vi "Stop Core.vi"(10 "final error code":i32, 11 "Device in":refnum<class "Device.lvclass">) -> (3 "Device out":refnum<class "Device.lvclass">)   [LabVIEW 2014, in "DAQ Device.lvlib" / "Device.lvclass"]
doc: "(<B>Filename</B>: Actor Framework.lvlib:Actor.lvclass:Stop Core.vi)\n\nDefines what the actor does before it stops. Use the <B>final error code</B> input to determine whether the actor shut down in response to an error.\n\nBy default, this method does nothing. A descendant class may override it to define behavior, such as shutting down any processes the actor initiated in its override of the Actor Core method."
uses:
  Device.lvclass
  SuperActor/SuperActor.lvclass/SuperActor.ctl
  Device.lvclass/Device.ctl
  SuperActor/Read Log Session.vi
  SuperActor/Read ID.vi
  <userlib>/_Session Fwk/Session - Root.lvclass
  Devices/Configurable Device/Configurable Device.lvclass
  SuperActor/SuperActor.lvclass
  Session APIs/Session Log/System Log.lvclass
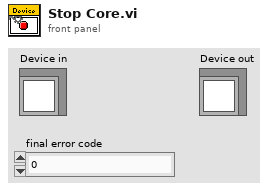
[diagram p1: front panel]
types:
  T1 = typedef "Session - Root.lvclass/Session Handle.ctl" = refnum<data-value>
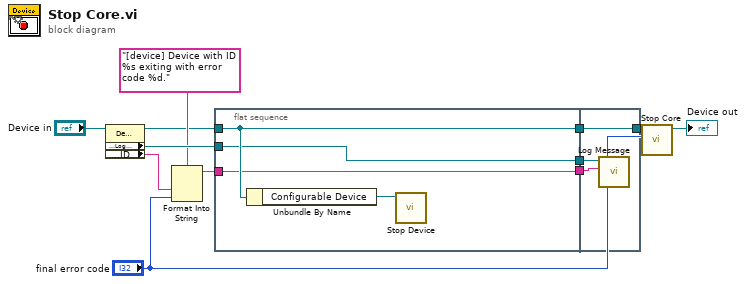
[diagram p0: block diagram]
diagram:
  n1 = property class="Device"(reference="Device in") -> (reference out=w5:refnum<class "Device.lvclass">, "Accessors:Log Session"=w10:T1, "Accessors:ID"=w7:string)  [unwired: 1 in, 1 out]
  n2 = Format Into String(format string="[device] Device with ID %s exiting with error code %d.", w7, "final error code") -> (resulting string=w6:string)  [unwired: 2 in, 1 out]
  n3 = flat-sequence {
    tunnel: w10 -> [w14]
    tunnel: w6 -> [w13]
    tunnel: w5 -> [w15]
    tunnel: [w15] -> w3
    tunnel: [w14] -> w2
    tunnel: [w13] -> w1
    tunnel: [w19] -> w4
    tunnel: w3 -> [w19]
    tunnel: w2 -> [w18]
    tunnel: w1 -> [w17]
    frame #0 {
      n4 = Unbundle By Name(w15) -> ("Configurable Device"=w16:refnum<class "Configurable Device.lvclass">)
      n5 = call-dynamic "Stop Device.vi"("Configurable Device in"=w16) -> ()  [unwired: 9 in, 2 out]
    }
    frame #1 {
      n6 = call "Log Message.vi"("MSG In"=w17, "session in"=w18) -> ()  [unwired: 8 in, 2 out]
    }
  }
  n7 = call-parent "Stop Core.vi"("final error code"="final error code", "Ex Nested in"=w4) -> ("Ex Nested out"=→"Device out":refnum<class "Device.lvclass">)  [unwired: 9 in]
